vi "Periodic Tasks.vi"(8 "error in":errorcluster) -> ()   [LabVIEW 2015]
doc: "This VI runs in parallel to other tasks. It can contain as many user-defined periodic loops as you need. These can carry out PID or other sorts of timed response."
uses:
  <vilib>/Rock Robotics/WPI/Utilities/WPI_GetSetVariantRefNum.vi
  Robot Global Data.vi
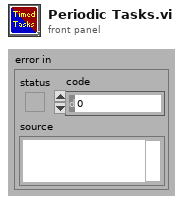
[diagram p1: front panel]
types:
  T1 = typedef "WPI_JoystickDevRef.ctl" = cluster{"Device":T2}
  T2 = typedef "WPI_JoystickDeviceEnum.ctl" = enum16{"USB 0", "USB 1", "USB 2", "USB 3", "USB 4", "USB 5"}
  T3 = cluster{"Axes[0]":dbl, "Axes[1]":dbl, "Axes[2]":dbl, "Axes[3]":dbl, "Axes[4]":dbl, "Axes[5]":dbl, "Axes[6]":dbl, "Axes[7]":dbl, "Axes[8]":dbl}
  T4 = cluster{"Buttons[0]":bool, "Buttons[1]":bool, "Buttons[2]":bool, "Buttons[3]":bool, "Buttons[4]":bool, "Buttons[5]":bool, "Buttons[6]":bool, "Buttons[7]":bool, "Buttons[8]":bool}
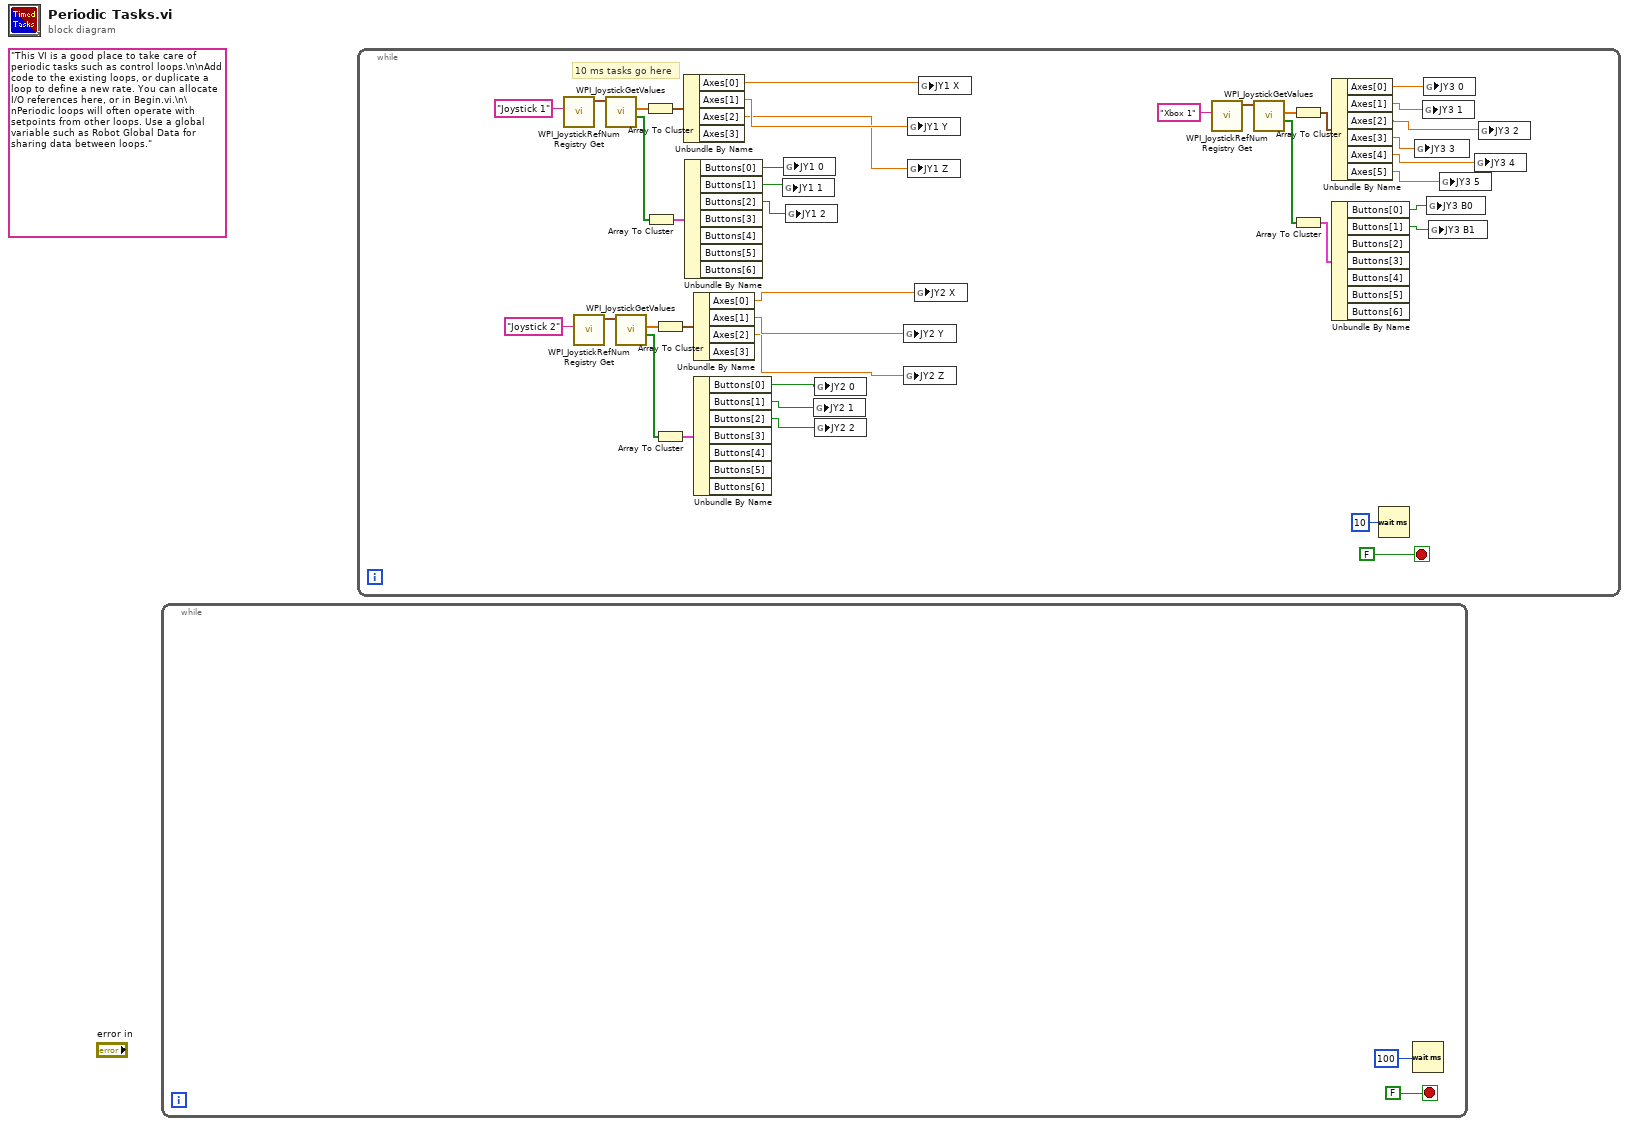
[diagram p0: block diagram]
diagram:
  (unwired) "This VI is a good place to take care of periodic tasks such as control loops.\n\nAdd code to the existing loops, or duplicate a loop to define a new rate. You can allocate I/O references here, or in Begin.vi.\n\nPeriodic loops will often operate with setpoints from other loops. Use a global variable such as Robot Global Data for sharing data between loops."
  n1 = while {
    stop <- FALSE stop-if-true
    n2 = Wait (ms)(milliseconds to wait=u32 100) -> ()  [unwired: 1 out]
  }
  n3 = while {
    stop <- FALSE stop-if-true
    # "10 ms tasks go here"
    n4 = call <vilib>:"WPI_JoystickRefNum Registry Get.vi"("refnum name"="Joystick 1") -> ("JoystickDevRef"=w41:T1)  [unwired: 1 in, 9 out]
    n5 = call <vilib>:"WPI_JoystickRefNum Registry Get.vi"("refnum name"="Joystick 2") -> ("JoystickDevRef"=w35:T1)  [unwired: 1 in, 9 out]
    n6 = call <vilib>:"WPI_JoystickGetValues.vi"("JoystickDevRef"=w41) -> ("Buttons"=w39:bool[], "Axes"=w38:dbl[])  [unwired: 6 in, 3 out]
    n7 = call <vilib>:"WPI_JoystickGetValues.vi"("JoystickDevRef"=w35) -> ("Buttons"=w33:bool[], "Axes"=w32:dbl[])  [unwired: 6 in, 3 out]
    n8 = Array To Cluster(array=w38) -> (cluster=w40:T3)
    n9 = Array To Cluster(array=w39) -> (cluster=w37:T4)
    n10 = Array To Cluster(array=w32) -> (cluster=w34:T3)
    n11 = Array To Cluster(array=w33) -> (cluster=w31:T4)
    n12 = Unbundle By Name(w40) -> ("Axes[0]"=w14:dbl, "Axes[1]"=w13:dbl, "Axes[2]"=w12:dbl)  [unwired: 1 out]
    n13 = Unbundle By Name(w37) -> ("Buttons[0]"=w30:bool, "Buttons[1]"=w29:bool, "Buttons[2]"=w4:bool)  [unwired: 4 out]
    n14 = Unbundle By Name(w34) -> ("Axes[0]"=w11:dbl, "Axes[1]"=w10:dbl, "Axes[2]"=w9:dbl)  [unwired: 1 out]
    n15 = Unbundle By Name(w31) -> ("Buttons[0]"=w28:bool, "Buttons[1]"=w25:bool, "Buttons[2]"=w3:bool)  [unwired: 4 out]
    n16 = global write "Robot Global Data.vi" "JY1 1"(w29) -> ()
    n17 = global write "Robot Global Data.vi" "JY1 0"(w30) -> ()
    n18 = global write "Robot Global Data.vi" "JY1 2"(w4) -> ()
    n19 = global write "Robot Global Data.vi" "JY2 1"(w25) -> ()
    n20 = global write "Robot Global Data.vi" "JY2 0"(w28) -> ()
    n21 = global write "Robot Global Data.vi" "JY2 2"(w3) -> ()
    n22 = global write "Robot Global Data.vi" "JY2 Y"(w10) -> ()
    n23 = global write "Robot Global Data.vi" "JY2 Z"(w9) -> ()
    n24 = global write "Robot Global Data.vi" "JY1 Y"(w13) -> ()
    n25 = global write "Robot Global Data.vi" "JY1 Z"(w12) -> ()
    n26 = global write "Robot Global Data.vi" "JY2 X"(w11) -> ()
    n27 = global write "Robot Global Data.vi" "JY1 X"(w14) -> ()
    n28 = call <vilib>:"WPI_JoystickRefNum Registry Get.vi"("refnum name"="Xbox 1") -> ("JoystickDevRef"=w23:T1)  [unwired: 1 in, 9 out]
    n29 = call <vilib>:"WPI_JoystickGetValues.vi"("JoystickDevRef"=w23) -> ("Buttons"=w21:bool[], "Axes"=w20:dbl[])  [unwired: 6 in, 3 out]
    n30 = Array To Cluster(array=w20) -> (cluster=w22:T3)
    n31 = Array To Cluster(array=w21) -> (cluster=w19:T4)
    n32 = Unbundle By Name(w22) -> ("Axes[0]"=w8:dbl, "Axes[1]"=w7:dbl, "Axes[2]"=w5:dbl, "Axes[3]"=w15:dbl, "Axes[4]"=w6:dbl, "Axes[5]"=w16:dbl)
    n33 = Unbundle By Name(w19) -> ("Buttons[0]"=w18:bool, "Buttons[1]"=w17:bool)  [unwired: 5 out]
    n34 = Wait (ms)(milliseconds to wait=u32 10) -> ()  [unwired: 1 out]
    n35 = global write "Robot Global Data.vi" "JY3 3"(w15) -> ()
    n36 = global write "Robot Global Data.vi" "JY3 1"(w7) -> ()
    n37 = global write "Robot Global Data.vi" "JY3 0"(w8) -> ()
    n38 = global write "Robot Global Data.vi" "JY3 B0"(w18) -> ()
    n39 = global write "Robot Global Data.vi" "JY3 B1"(w17) -> ()
    n40 = global write "Robot Global Data.vi" "JY3 5"(w16) -> ()
    n41 = global write "Robot Global Data.vi" "JY3 4"(w6) -> ()
    n42 = global write "Robot Global Data.vi" "JY3 2"(w5) -> ()
  }
